vi "Find Duplicate.vi"(10 "Array":string[](array[string])) -> (1 "Index 2":i32, 2 "Index 1":i32, 3 "Duplicate":bool)   [LabVIEW 2014, in "Shared Memory configuration.lvclass"]
uses:
  Shared Memory configuration.lvclass
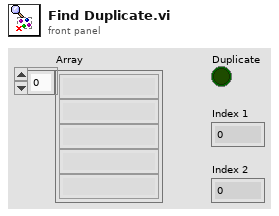
[diagram p1: front panel]
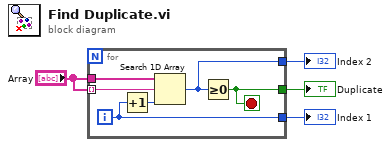
[diagram p0: block diagram]
diagram:
  n1 = for {
    tunnel: "Array" -> [w9] mode=indexing
    tunnel: "Array" -> [w10]
    tunnel: [w8] -> w3
    tunnel: [w5] -> w2
    tunnel: [w7] -> w1
    i -> [w5]
    stop <- w8 stop-if-true
    n2 = Increment(x=w5) -> (x+1=w6:i32)
    n3 = Search 1D Array(1D array=w10, element=w9, start index (0)=w6) -> (index of element=w7:i32)
    n4 = Greater Or Equal To 0?(x=w7) -> (x >= 0?=w8:bool)
  }
  "Duplicate" <- w3
  "Index 1" <- w2
  "Index 2" <- w1
